vi "Write Array.vi"(8 "Error In":errorcluster, 10 "Elements Count":u32, 11 "Writer In":refnum<class "Writer.lvclass">) -> (0 "Error Out":errorcluster, 3 "Writer Out":refnum<class "Writer.lvclass">)   [LabVIEW 2019, in "LabPack.lvlib" / "Writer.lvclass"]
uses:
  Writer.lvclass
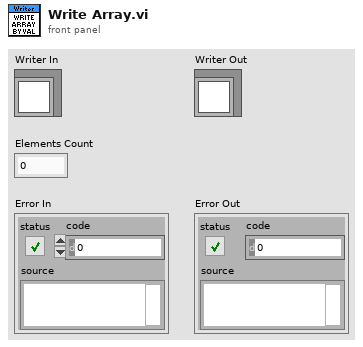
[diagram p1: front panel]
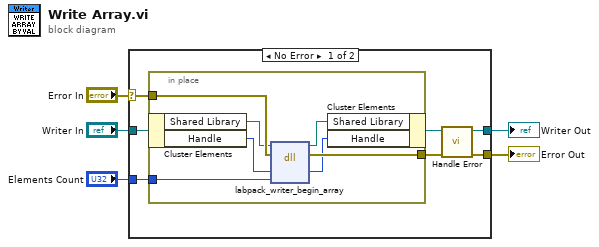
[diagram p0: block diagram]
diagram:
  n1 = case shown="No Error" "Error In" {
    selector: "Error In" -> [w12 w21]
    tunnel: [w7 w21] -> w4
    tunnel: "Writer In" -> [w11 w20]
    tunnel: [w9 w20] -> w2
    tunnel: "Elements Count" -> [w6 _]
    frame No Error {
      n2 = in-place {
        in-place-border: w12 -> [w19]
        in-place-border: [w18] -> w8
        in-place-border: w6 -> [w13]
        n3 = in-place-cluster #1(w11) -> ("Shared Library"=w17:path, "Handle"=w15:u64)
        n4 = dll-call lib="D:/Users/cfield/Code/MessagePack/LabPack/LabVIEW/trunk/src/LabPack/Private/labpack-x64.dll" fn="labpack_writer_begin_array"(path in=w17, error in=w19, "writer"=w15, "count"=w13) -> (path out=w16:path, error out=w18:errorcluster, "writer"=w14:u64)  [unwired: 3 in]
        n5 = in-place-cluster #1("Shared Library"=w16, "Handle"=w14) -> (w10:refnum<class "Writer.lvclass">)
      }
      n6 = call "Handle Error.vi"("Error In"=w8, "Writer In"=w10) -> ("Error Out"=w7:errorcluster, "Writer Out"=w9:refnum<class "Writer.lvclass">)  [unwired: 8 in]
    }
    frame Error {
    }
  }
  "Error Out" <- w4
  "Writer Out" <- w2
